vi "Value Updates.vi"(11 "DaqControl in":T1) -> (3 "DaqControl out":T1)   [LabVIEW 2020, in "VolatusDaq.lvlib" / "DaqControl.lvclass"]
uses:
  DaqControl.lvclass
  Loop Data.ctl
  Volatus/Event API/EventAPI.lvclass
  Volatus/DataHandlerAPI/DataHandlerAPI.lvclass
  Sequence Action.ctl
  Seq Action Type.ctl
  Value Update.ctl
  Seq Cmd.ctl
  Seq Cmd Type.ctl
  Signal Type.ctl
  DaqControl.lvclass/DaqControl.ctl
  VolatusDaq.lvlib
  Sequence.ctl
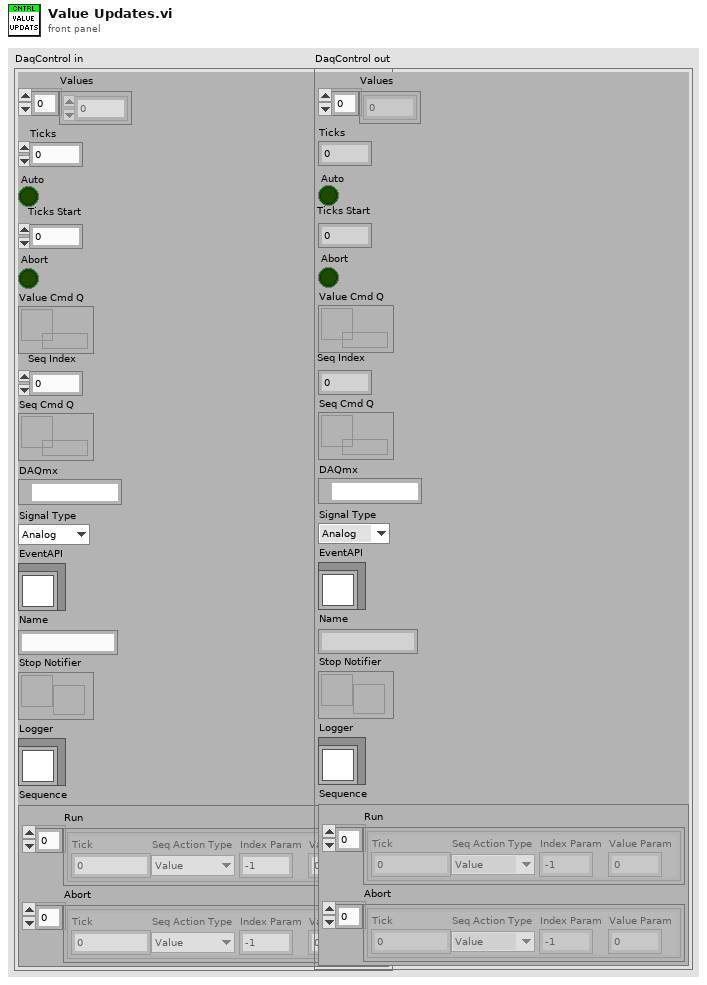
[diagram p1: front panel]
types:
  T1 = typedef "VolatusDaq.lvlib/DaqControl.lvclass/Loop Data.ctl" = cluster{"Values":dbl[], "Ticks":u32, "Auto":bool, "Ticks Start":u32, "Abort":bool, "Value Cmd Q":refnum<queue>, "Seq Index":i32, "Seq Cmd Q":refnum<queue>, "DAQmx":refnum<k21>, "Signal Type":T2, "EventAPI":refnum<class "EventAPI.lvclass">, "Name":string, "Stop Notifier":refnum<notifier>, "Logger":refnum<class "DataHandlerAPI.lvclass">, "Sequence":T3}
  T2 = typedef "VolatusDaq.lvlib/Signal Type.ctl" = enum16{"Analog", "Digital"}
  T3 = typedef "VolatusDaq.lvlib/Sequence.ctl" = cluster{"Run":T4[], "Abort":T4[]}
  T4 = typedef "VolatusDaq.lvlib/Sequence Action.ctl" = cluster{"Tick":u32, "Seq Action Type":T5, "Index Param":i32, "Value Param":dbl}
  T5 = typedef "VolatusDaq.lvlib/Seq Action Type.ctl" = enum16{"Value", "Stop"}
  T6 = typedef "VolatusDaq.lvlib/DaqControl.lvclass/Value Update.ctl" = cluster{"Index":i32, "Value":dbl}
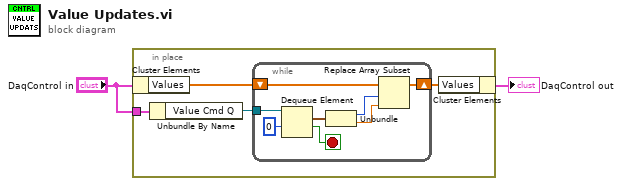
[diagram p0: block diagram]
diagram:
  n1 = in-place {
    in-place-border: "DaqControl in" -> [w6]
    n2 = in-place-cluster #1("DaqControl in") -> ("Values"=w5:dbl[])
    n3 = Unbundle By Name(w6) -> ("Value Cmd Q"=w4:refnum<queue>)
    n4 = while {
      shift-right: [w7] -> w3
      shift-left: w5 -> [w11]
      tunnel: w4 -> [w14]
      stop <- w12 stop-if-true
      n5 = Dequeue Element(queue=w14, timeout in ms (-1)=0) -> (element=w10:T6, timed out?=w12:bool)  [unwired: 1 in, 2 out]
      n6 = Unbundle(w10) -> ("Index"=w9:i32, "Value"=w8:dbl)
      n7 = Replace Array Subset(array=w11, new element=w8, index=w9) -> (w7:dbl[])
    }
    n8 = in-place-cluster #1("Values"=w3) -> (→"DaqControl out":T1)
  }
